vi "test.vi"() -> ()   [LabVIEW 2018]
uses:
  <vilib>/Analysis/4window.llb/Gaussian Window (DBL).vi
  <vilib>/Analysis/NI_AALPro.lvlib
panel:
  out "FR Graph":dbl[][](graph)
  out "FIR Graph":dbl[][](graph)
  in  "Native FR":dbl[](array[numeric])=[1.0, 1.0, 1.0, 0.0, 0.0, 0.0, 0.0, 0.0]
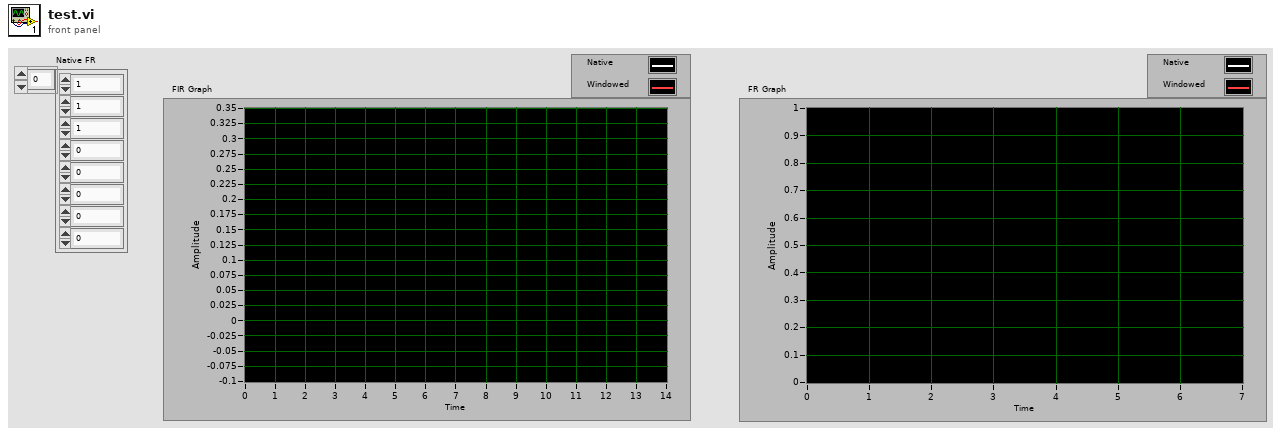
[diagram p1: front panel]
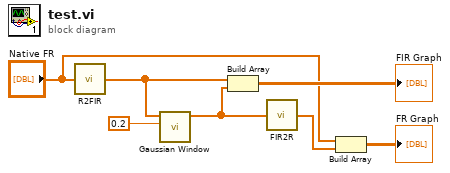
[diagram p0: block diagram]
diagram:
  n1 = call "R2FIR.vi"("Frequency"="Native FR") -> ("FIR coefficients"=w4:dbl[])  [unwired: 4 in]
  n2 = call-poly <vilib>:"Gaussian Window.vi"("standard deviation"=0.2, "X"=w4) -> ("Windowed X"=w5:dbl[])  [unwired: 8 in, 1 out]
  n3 = Build Array(w4, w5) -> (→"FIR Graph":dbl[][])
  n4 = call "FIR2R.vi"("FIR coefficients"=w5) -> ("Frequency"=w2:dbl[])
  n5 = Build Array("Native FR", w2) -> (→"FR Graph":dbl[][])
